vi "RH_Relays_ConnectDisconnect.vi"(7 "relay action (Close Relay)":T1=21 items=["Open Relay"=20, "Close Relay"=21], 8 "error in":errorcluster, 9 "settling (s)":dbl, 10 "relay names":string, 11 "Relays Session In":refnum<k15>) -> (0 "error out":errorcluster, 3 "Relays Session Out":refnum<k15>)   [LabVIEW 2023, in "ResourceHandling.lvlib"]
doc: "Connect / Disconnect the relasy channels"
uses:
  ResourceHandling.lvlib
  <instrlib>/niSwitch/niSwitch.llb/niSwitch Relay Action.ctl
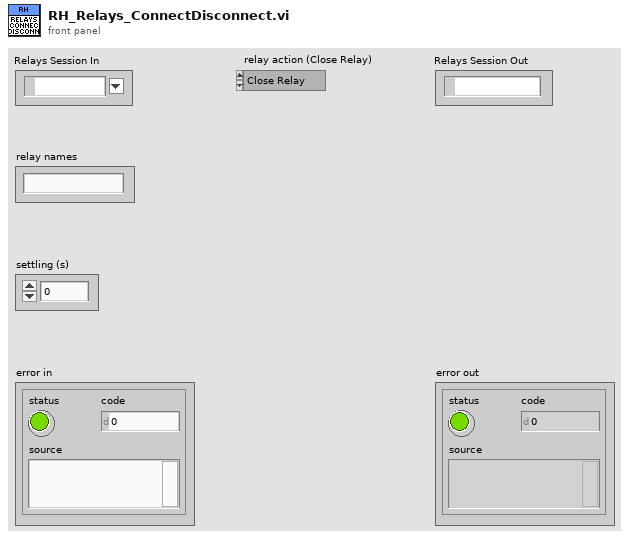
[diagram p1: front panel]
types:
  T1 = typedef "niSwitch Relay Action.ctl" = i32
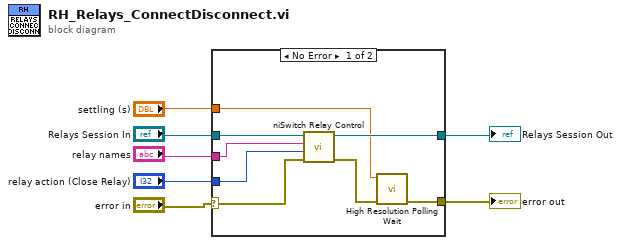
[diagram p0: block diagram]
diagram:
  n1 = case shown="No Error" "error in" {
    selector: "error in" -> [w14 w17]
    tunnel: "Relays Session In" -> [w15 w16]
    tunnel: [w9 w16] -> w5
    tunnel: [w10 w17] -> w4
    tunnel: "relay action (Close Relay)" -> [w13 _]
    tunnel: "relay names" -> [w12 _]
    tunnel: "settling (s)" -> [w8 _]
    frame No Error {
      n2 = call <instrlib>:"niSwitch Relay Control.vi"("error in (no error)"=w14, "relay action (Close Relay)"=w13, "relay names"=w12, "instrument handle"=w15) -> ("error out"=w11:errorcluster, "instrument handle out"=w9:refnum<k15>)  [unwired: 6 in]
      n3 = call <vilib>:"High Resolution Polling Wait.vi"("error in (no error)"=w11, "seconds to wait"=w8) -> ("error out"=w10:errorcluster)  [unwired: 9 in]
    }
    frame Error {
    }
  }
  "error out" <- w4
  "Relays Session Out" <- w5
